vi "Test_API_DelayedShutdown_PostCloseLogAvailable.vi"(8 "error in (no error)":errorcluster, 11 "TestCase in":refnum<class "TestLocalLogInstance.lvclass">) -> (0 "error out":errorcluster, 3 "TestCase out":refnum<class "TestLocalLogInstance.lvclass">)   [LabVIEW 2017, in "TestLocalLogInstance.lvclass"]
uses:
  TestLocalLogInstance.lvclass
  Source/Composed Log/LoggerReference/LoggerReference.lvclass/LoggerReference.ctl
  8950b9ed-0ce6-4bc0-9a08-7d781de0ef0c.vi
  Source/Composed Log/LoggerReference/Return Aggregate Queues.vi
  Source/Composed Log/LoggerReference/Add Aggregate Log.vi
  8950b9ed-0ce6-4bc0-9a08-7d781de0ef0c.vi/c09e0496-24ef-4e3a-bb9f-f98b490e17c6.vi
  Source/Composed Log/LoggerReference/Log.vi
  Source/Composed Log/LoggerReference/Send Add Sink.vi
  Source/Composed Log/LoggerReference/Remove Stale Logs.vi
  Source/LVQueue Sink/LVQueue Sink.lvclass
  C:/CS/Internal/LabVIEW/Logger/Source/Composed Log/Log Sink/Log Sink.lvclass
  Source/Composed Log/Application Logger/Launch Worker Loop.vi
  Source/Composed Log/LoggerReference/Initialize Logger Instance.vi
  Source/Composed Log/LoggerReference/LoggerReference.lvclass
  Source/Composed Log/IErrorFormat/IErrorFormat.lvclass
  Source/Composed Log/Log Sink/Log Sink.lvclass
  <vilib>/addons/_JKI Toolkits/VI Tester/TestCase.llb/TestCase.lvclass
  C:/Program Files (x86)/National Instruments/LabVIEW 2017/vi.lib/addons/_JKI Toolkits/VI Tester/TestCase.llb/TestCase.lvclass
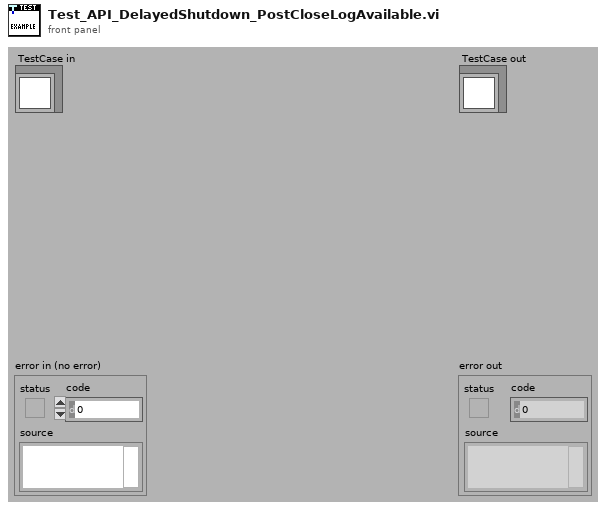
[diagram p1: front panel]
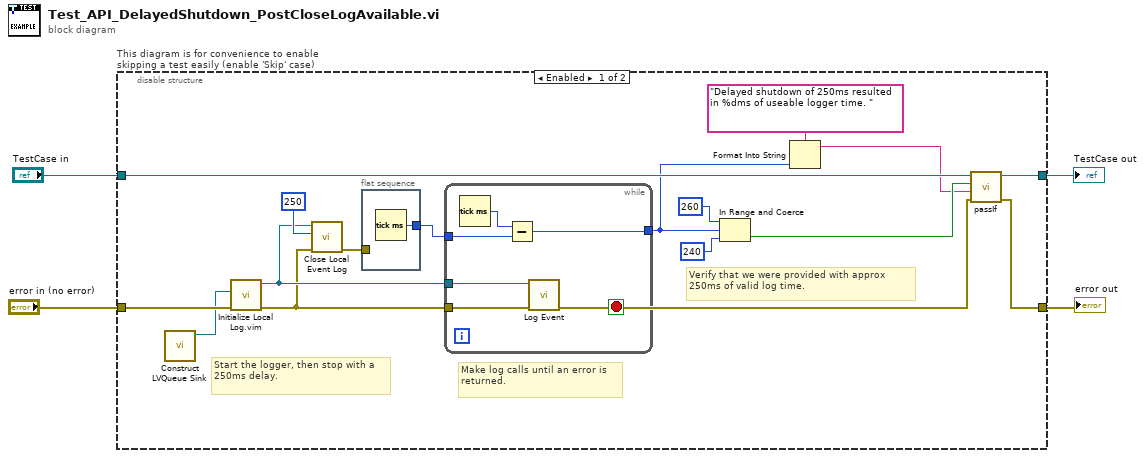
[diagram p0: block diagram]
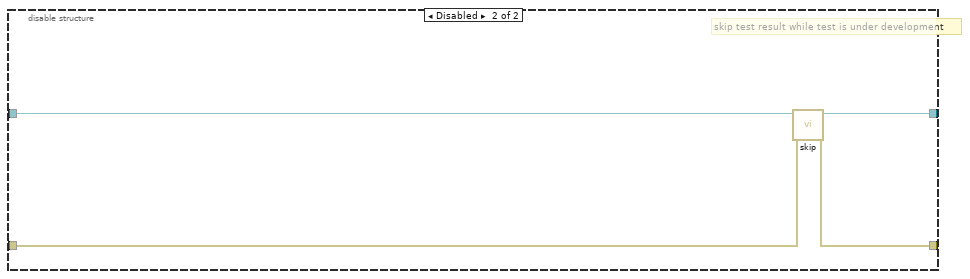
[diagram p2: hidden frame]
diagram:
  n1 = disable-structure "This diagram is for convenience to enable skipping a test easily (enable 'Skip' case)" shown="Enabled" {
    disable-tunnel: "TestCase in" -> [w19 w31]
    disable-tunnel: [w18 w29] -> w1
    disable-tunnel: [w17 w30] -> w3
    disable-tunnel: "error in (no error)" -> [w10 w28]
    frame Enabled {
      # "Verify that we were provided with approx 250ms of valid log time."
      # "Make log calls until an error is returned."
      # "Start the logger, then stop with a 250ms delay."
      n2 = call "Construct LVQueue Sink.vi"() -> ("LVQueue Sink out"=w8:refnum<class "LVQueue Sink.lvclass">)  [unwired: 10 in, 1 out]
      n3 = call "Initialize Local Log.vim"("error in (no error)"=w10, "Startup Sink(s)"=w8) -> ("error out"=w5:errorcluster, "Log Instance Reference"=w6:refnum<class "LoggerReference.lvclass">)  [unwired: 7 in, 1 out]
      n4 = call "Close Local Event Log.vi"("error in (no error)"=w5, "Deferred Close Time (0 ms)"=u32 250 ("Deferred Close Time (ms)"), "Log Instance"=w6) -> ("error out"=w9:errorcluster)  [unwired: 8 in]
      n5 = flat-sequence {
        tunnel: w9 -> [_]
        tunnel: [w21] -> w20
        frame #0 {
          n6 = Tick Count (ms)() -> (millisecond timer value=w21:u32)
        }
      }
      n7 = while {
        tunnel: w5 -> [w25]
        tunnel: w20 -> [w26]
        tunnel: [w23] -> w14
        tunnel: w6 -> [w22]
        stop <- w24 stop-if-true
        n8 = Tick Count (ms)() -> (millisecond timer value=w27:u32)
        n9 = Subtract(x=w27, y=w26) -> (x-y=w23:u32)
        n10 = call "Log Event.vi"("error in (no error)"=w25, "Log Instance"=w22) -> ("error out"=w24:errorcluster)  [unwired: 8 in, 1 out]
      }
      n11 = In Range and Coerce(upper limit=u32 260 ("lower limit"), x=w14, lower limit=u32 240 ("upper limit")) -> (In Range?=w16:bool)  [unwired: 1 out]
      n12 = Format Into String(format string="Delayed shutdown of 250ms resulted in %dms of useable logger time. ", w14) -> (resulting string=w13:string)  [unwired: 2 in, 1 out]
      n13 = call-dynamic "passIf.vi"("error in (no error)"=w5, "message (\"\")"=w13, "pass"=w16, "TestCase in"=w19) -> ("error out"=w17:errorcluster, "TestCase out"=w18:refnum<class "TestLocalLogInstance.lvclass">)  [unwired: 6 in]
    }
    frame Disabled {
      # "skip test result while test is under development"
      n14 = call <vilib>:"skip.vi"("error in (no error)"=w28, "TestCase in"=w31) -> ("error out"=w30:errorcluster, "TestCase out"=w29:refnum<class "TestLocalLogInstance.lvclass">)  [unwired: 8 in]
    }
  }
  "error out" <- w3
  "TestCase out" <- w1
